vi "Send Int to ROS.vi"() -> ()   [LabVIEW 2018]
uses:
  <vilib>/RTI DDS Toolkit/Types/RTI DDS Advanced Writer Configuration.ctl
  <vilib>/RTI DDS Toolkit/VIs/AdvancedCreateWriter_NumI32.vi
  <vilib>/RTI DDS Toolkit/VIs/Write_NumI32.vi
  <vilib>/RTI DDS Toolkit/Library/LVDDS_library.lvlib
panel:
  out "to ROS":i32
  in  "stop":bool
  in  "error in (no error)":errorcluster
  in  "Advanced Writer Configuration":T1={"typeName"="std_msgs::msg::dds_::Int32_", "keyName"="", "domainParticipantQoSProfile"="", "dataWriterQoSProfile"="", "forceArrayMapping?"=FALSE, "forceUnboundedString?"=FALSE}
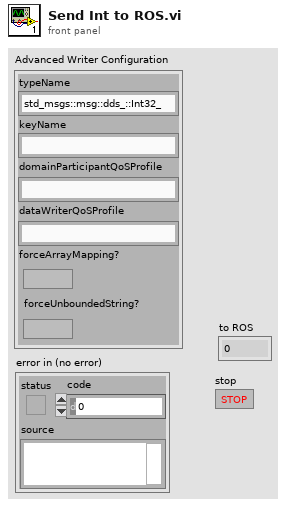
[diagram p1: front panel]
types:
  T1 = typedef "LVDDS_library.lvlib/RTI DDS Advanced Writer Configuration.ctl" = cluster{"typeName":string, "keyName":string, "domainParticipantQoSProfile":string, "dataWriterQoSProfile":string, "forceArrayMapping?":bool, "forceUnboundedString?":bool}
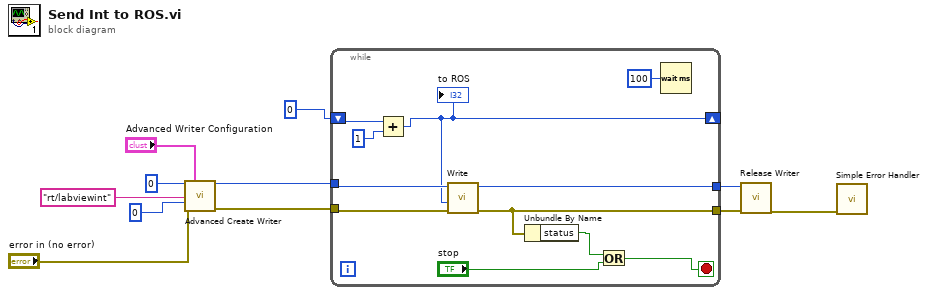
[diagram p0: block diagram]
diagram:
  n1 = call-poly <vilib>:"Advanced Create Writer.vi"("Domain Id"=u32 0, "Advanced Writer Configuration"="Advanced Writer Configuration", "Topic Name"="rt/labviewint", "Data Type"=0, "error in (no error)"="error in (no error)") -> ("DDS Object Ref"=w5:u64, "error out"=w4:errorcluster)  [unwired: 9 in]
  n2 = while {
    shift-right: [w17] -> _
    shift-left: 0 -> [w21]
    tunnel: w5 -> [w19]
    tunnel: w4 -> [w18]
    tunnel: [w16] -> w3
    tunnel: [w15] -> w2
    stop <- w12 stop-if-true
    n3 = Add(x=w21, y=1) -> (x+y=w17:i32)
    "to ROS" <- w17
    n4 = call-poly <vilib>:"Write.vi"("error in (no error)"=w18, "Data"=w17, "DDS Object Ref in"=w19) -> ("error out"=w15:errorcluster, "DDS Object Ref out"=w16:u64)  [unwired: 7 in]
    n5 = Unbundle By Name "Unbundle By Name"(w15) -> ("status"=w14:bool)
    n6 = Or(x=w14, y="stop") -> (x .or. y?=w12:bool)
    n7 = Wait (ms)(milliseconds to wait=u32 100) -> ()  [unwired: 1 out]
  }
  n8 = call <vilib>:"Release Writer.vi"("error in (no error)"=w2, "DDS Object Ref"=w3) -> ("error out"=w1:errorcluster)  [unwired: 9 in]
  n9 = call <vilib>:"Simple Error Handler.vi"("error in (no error)"=w1) -> ()  [unwired: 4 in, 5 out]
